vi "Setup UI temp.vi"(8 "error in (no error)":errorcluster, 10 "Set UI to input? (F)":bool, 11 "PC Reader.lvclass":refnum<class "PC Reader.lvclass">) -> (0 "error out":errorcluster, 3 "PC Reader out":refnum<class "PC Reader.lvclass">)   [LabVIEW 2009, in "PC Reader.lvclass"]
doc: "Setup UI (re)constructs an object -- populates its member data -- from a front panel the user can see. The VI should be as simple as possible so that a UI loop can poll it continuously for updates. \n\nThe VI is designed to be used as a subPanel within another VI. Wire true to \"Set UI to input\" only on the first call, just after inserting this VI into a subPanel, to populate its controls with the class's current values.\n\nSetup UI is distinct from the class constructor. Class constructors are not polymorphic, yet configure dialogs need to configure objects without knowing their type -- and polymorphism is the necessary solution. Thus, Setup UI is a polymorphic class constructor. This continously polled \"Setup UI\" concept is a kludge: a better idea would be an XControl, but those require a steeper learning curve."
uses:
  PC Reader.lvclass
  PC Reader.lvclass/PC Reader.ctl
panel:
  in  "template: Ch A sweep":bool
  in  "template: Ch A/B split":bool
  in  "template: continuous scan":bool
  in  "Gate B Ref":enum16{"t=0", "t=T/4", "t=T/2", "t=3T/4"}(ring)
  in  "Gate A Ref":enum16{"t=0", "t=T/4", "t=T/2", "t=3T/4"}(ring)
  out "Gate B Delay Actual":dbl[unit]
  out "Gate A Delay Actual":dbl[unit]
  in  "start vs mid. of gate":bool caption="Delays measured to"
  in  "Gate B %":dbl
  in  "Gate A %":dbl
  in  "time vs percent":bool caption="Width in"
  out "Gate B Mode":enum16{"CW", "Fixed", "Scan"}(ring)
  out "Gate A Mode":enum16{"CW", "Fixed", "Scan"}(ring)
  in  "Gate B Width":dbl[unit]
  in  "Gate B Delay":dbl[unit]
  in  "Gate A Delay":dbl[unit]
  in  "Gate A Width":dbl[unit]
  in  "Ext. Trigger?":bool
  in  "Ext. Trig. Freq.":dbl[unit]
  in  "Count Time":dbl[unit] format="%#_4g"
  in  "Send first pt to PC":bool
  in  "indAw?":bool
  in  "indAd?":bool
  in  "indBw?":bool
  in  "indBd?":bool
  # "Photon Counter Setup"
  # "Track ind.var.?\n(assumes in ns)"
  # "(PEM = 42.0762 kHz)"
  # "(If tracking, these times represent \nthe values for the first pt.)"
  # "PURE VIRTUAL\nMETHOD CALLED!"
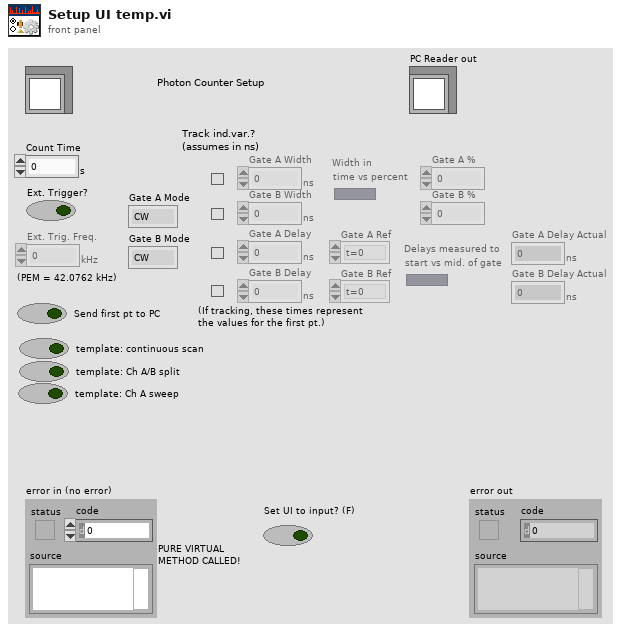
[diagram p1: front panel]
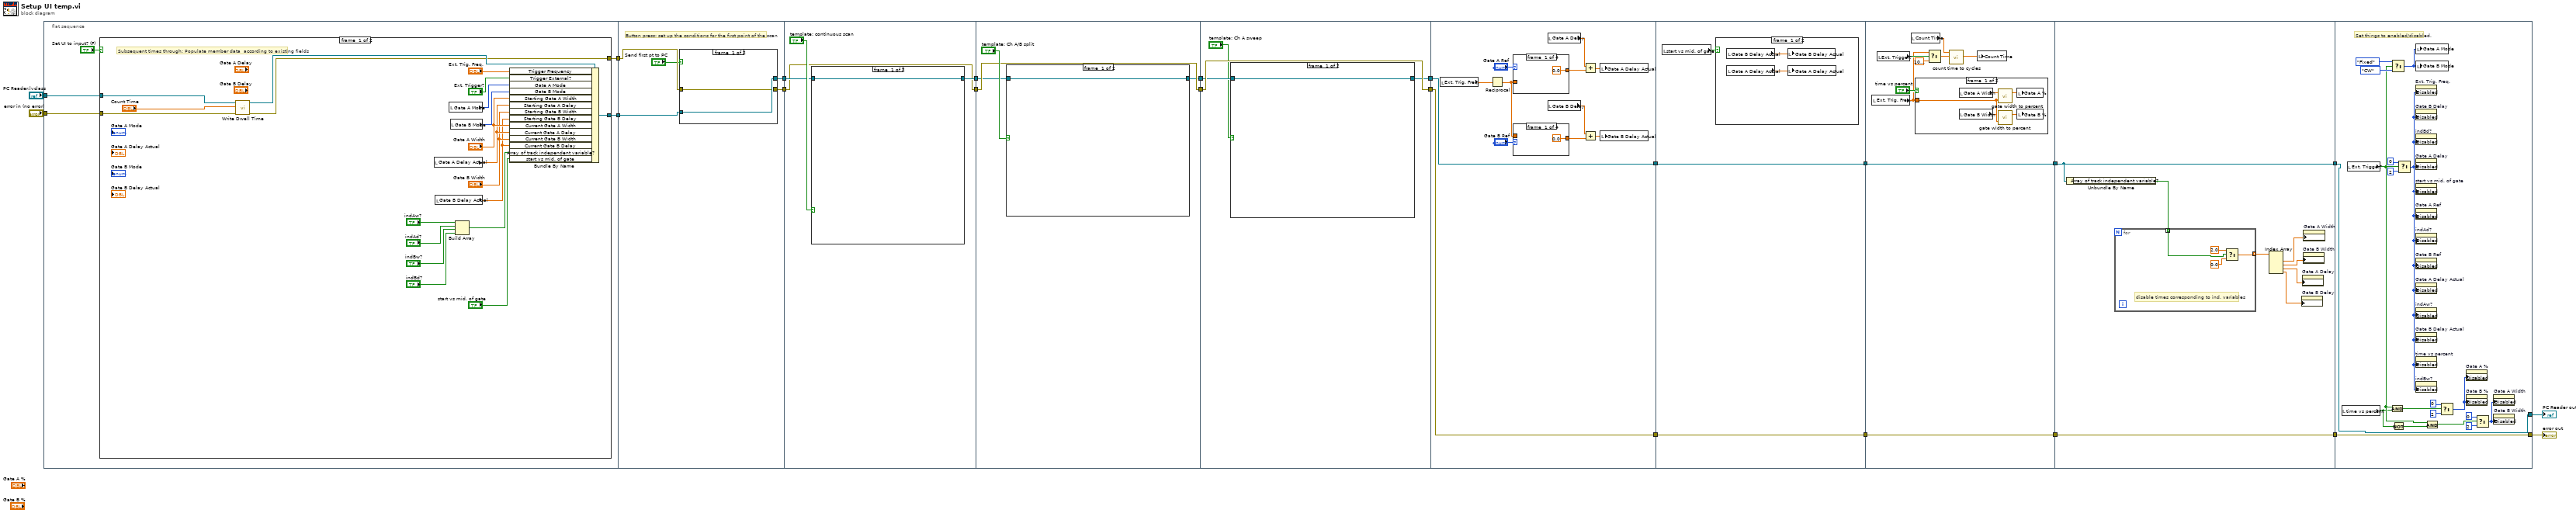
[diagram p0: block diagram]
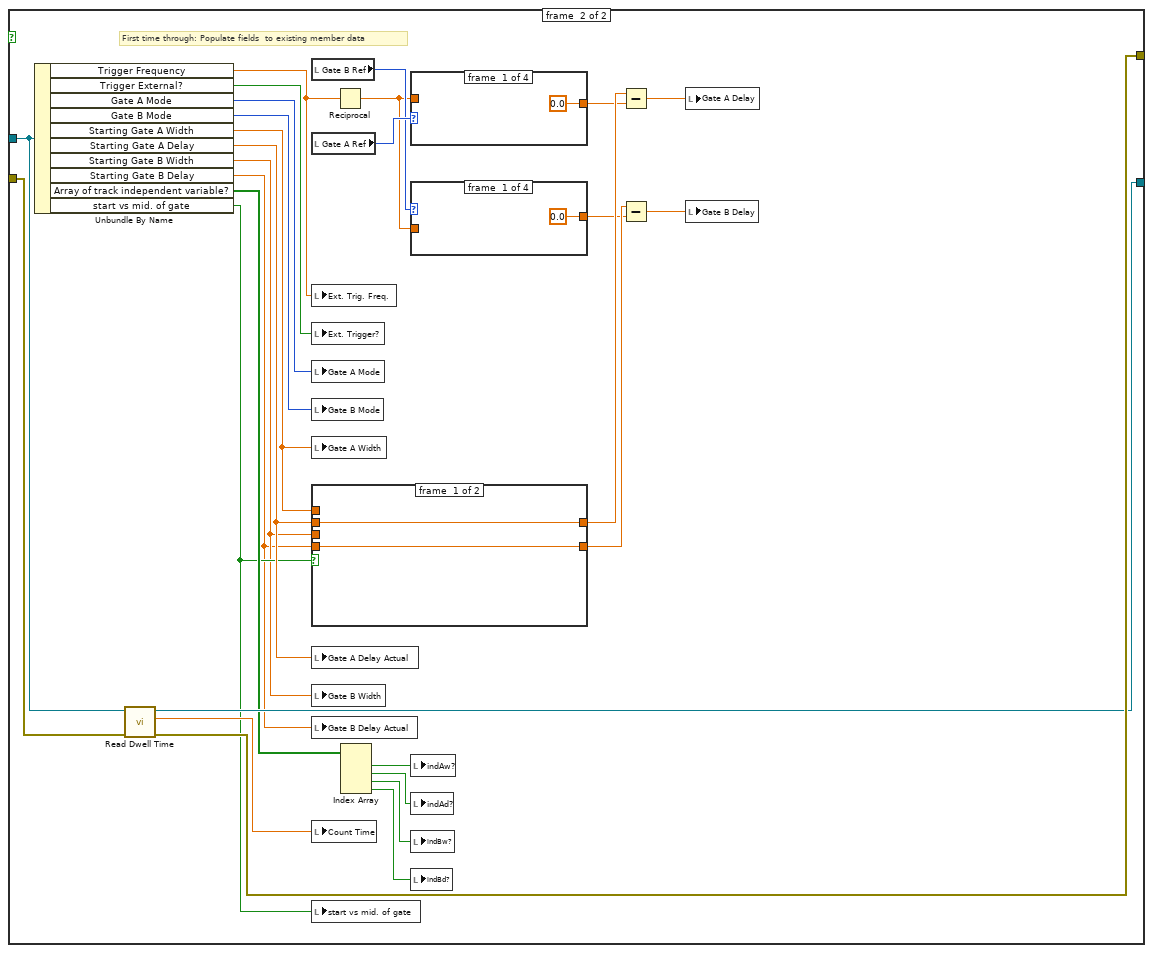
[diagram p2: hidden frame]
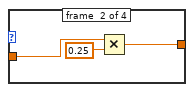
[diagram p3: hidden frame]
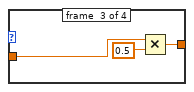
[diagram p4: hidden frame]
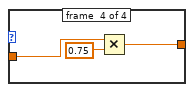
[diagram p5: hidden frame]
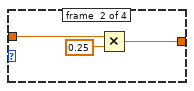
[diagram p6: hidden frame]
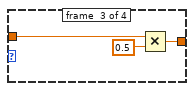
[diagram p7: hidden frame]
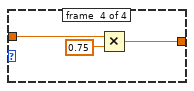
[diagram p8: hidden frame]
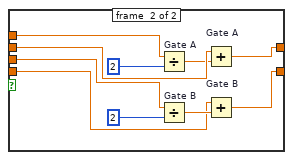
[diagram p9: hidden frame]
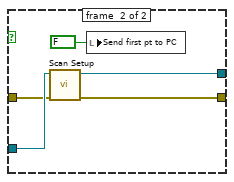
[diagram p10: hidden frame]
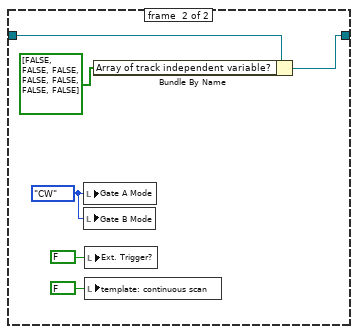
[diagram p11: hidden frame]
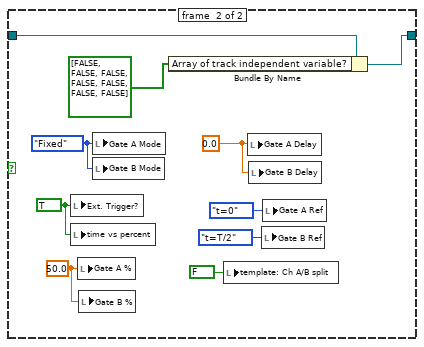
[diagram p12: hidden frame]
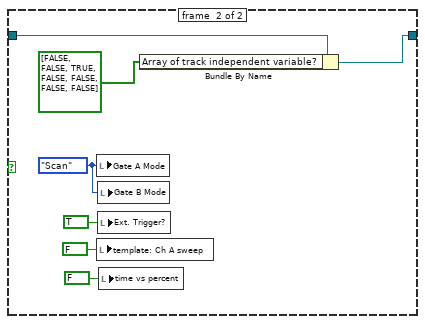
[diagram p13: hidden frame]
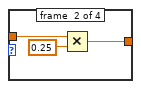
[diagram p14: hidden frame]
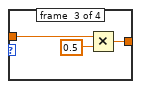
[diagram p15: hidden frame]
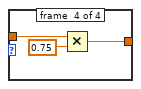
[diagram p16: hidden frame]
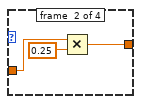
[diagram p17: hidden frame]
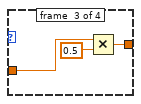
[diagram p18: hidden frame]
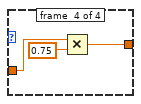
[diagram p19: hidden frame]
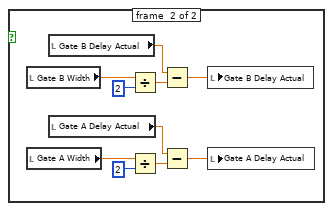
[diagram p20: hidden frame]
diagram:
  n1 = flat-sequence {
    tunnel: "error in (no error)" -> [w24]
    tunnel: [w27] -> w16
    tunnel: [w23] -> w15
    tunnel: "PC Reader.lvclass" -> [w25]
    tunnel: w16 -> [w112]
    tunnel: w15 -> [w111]
    tunnel: [w110] -> w14
    tunnel: [w108] -> w13
    tunnel: w14 -> [w120]
    tunnel: w13 -> [w122]
    tunnel: [w121] -> w12
    tunnel: [w120] -> w11
    tunnel: w12 -> [w132]
    tunnel: [w131] -> w10
    tunnel: w11 -> [w133]
    tunnel: [w133] -> w8
    tunnel: w10 -> [w148]
    tunnel: [w147] -> w9
    tunnel: w8 -> [w149]
    tunnel: [w149] -> w7
    tunnel: [w169] -> w19
    tunnel: [w168] -> w18
    tunnel: w9 -> [w168]
    tunnel: w7 -> [w169]
    tunnel: w19 -> [w192]
    tunnel: [w192] -> w21
    tunnel: w18 -> [w191]
    tunnel: [w191] -> w20
    tunnel: w21 -> [w213]
    tunnel: [w213] -> w6
    tunnel: w20 -> [w212]
    tunnel: [w212] -> w4
    tunnel: w6 -> [w231]
    tunnel: [w231] -> w5
    tunnel: w4 -> [w225]
    tunnel: [w225] -> w3
    tunnel: w5 -> [w237]
    tunnel: w3 -> [w236]
    tunnel: [w237] -> w2
    tunnel: [w236] -> w1
    frame #0 {
      n2 = case shown="True" "Set UI to input? (F)" {
        tunnel: [w39 w66] -> w27
        tunnel: w25 -> [w40 w67]
        tunnel: [w36 w68] -> w23
        tunnel: w24 -> [w35 w69]
        frame #0 {
          # "Subsequent times through: Populate member data  according to existing fields"
          n3 = call-dynamic "Write Dwell Time.vi"("error in (no error)"=w35, "Dwell Time"="Count Time", "Reader.lvclass in"=w40) -> ("error out"=w36:errorcluster, "Reader.lvclass out"=w38:refnum<class "PC Reader.lvclass">)  [unwired: 7 out]
          n4 = local read "Gate A Delay Actual"() -> (w32:dbl[unit])
          n5 = local read "Gate B Delay Actual"() -> (w30:dbl[unit])
          n6 = local read "Gate A Mode"() -> (w41:enum16{"CW", "Fixed", "Scan"})
          n7 = local read "Gate B Mode"() -> (w34:enum16{"CW", "Fixed", "Scan"})
          n8 = Build Array("indAw?", "indAd?", "indBw?", "indBd?") -> (w29:bool[])
          n9 = Bundle By Name(cluster=w38, "Trigger Frequency"="Ext. Trig. Freq.", "Trigger External?"="Ext. Trigger?", "Gate A Mode"=w41, "Gate B Mode"=w34, "Starting Gate A Width"="Gate A Width", "Starting Gate A Delay"=w32, "Starting Gate B Width"="Gate B Width", "Starting Gate B Delay"=w30, "Current Gate A Width"="Gate A Width", "Current Gate A Delay"=w32, "Current Gate B Width"="Gate B Width", "Current Gate B Delay"=w30, "Array of track independent variable?"=w29, "start vs mid. of gate"="start vs mid. of gate") -> (w39:refnum<class "PC Reader.lvclass">)
        }
        frame #1 {
          # "First time through: Populate fields  to existing member data"
          n10 = Unbundle By Name(w67) -> ("Trigger Frequency"=w62:dbl[unit], "Trigger External?"=w71:bool, "Gate A Mode"=w70:u16, "Gate B Mode"=w56:u16, "Starting Gate A Width"=w54:dbl[unit], "Starting Gate A Delay"=w55:dbl[unit], "Starting Gate B Width"=w51:dbl[unit], "Starting Gate B Delay"=w50:dbl[unit], "Array of track independent variable?"=w53:bool[], "start vs mid. of gate"=w52:bool)
          n11 = call-dynamic "Read Dwell Time.vi"("error in (no error)"=w69, "Reader.lvclass in"=w67) -> ("error out"=w68:errorcluster, "Dwell Time"=w65:dbl[unit], "Reader.lvclass out"=w66:refnum<class "PC Reader.lvclass">)  [unwired: 7 out]
          n12 = local read "Gate B Ref"() -> (w63:enum16{"t=0", "t=T/4", "t=T/2", "t=3T/4"})
          n13 = local read "Gate A Ref"() -> (w64:enum16{"t=0", "t=T/4", "t=T/2", "t=3T/4"})
          n14 = local write "Ext. Trig. Freq."(w62) -> ()
          n15 = local write "Ext. Trigger?"(w71) -> ()
          n16 = local write "Gate A Mode"(w70) -> ()
          n17 = local write "Gate B Mode"(w56) -> ()
          n18 = local write "Gate A Width"(w54) -> ()
          n19 = case shown="False" w52 {
            tunnel: [w97 w101] -> w60
            tunnel: w55 -> [w97 w105]
            tunnel: [w96 w100] -> w57
            tunnel: w54 -> [_ w102]
            tunnel: w51 -> [_ w99]
            tunnel: w50 -> [w96 w98]
            frame #0 {
            }
            frame #1 {
              n20 = Divide "Gate A"(x=w102, y=2) -> (x/y=w104:dbl[unit])
              n21 = Divide "Gate B"(x=w99, y=2) -> (x/y=w103:dbl[unit])
              n22 = Add "Gate A"(x=w105, y=w104) -> (x+y=w101:dbl[unit])
              n23 = Add "Gate B"(x=w98, y=w103) -> (x+y=w100:dbl[unit])
            }
          }
          n24 = local write "Gate A Delay Actual"(w55) -> ()
          n25 = local write "Gate B Width"(w51) -> ()
          n26 = local write "Gate B Delay Actual"(w50) -> ()
          n27 = local write "Count Time"(w65) -> ()
          n28 = local write "start vs mid. of gate"(w52) -> ()
          n29 = Reciprocal(x=w62) -> (1/x=w61:dbl[unit])
          n30 = Index Array(array=w53) -> (element #1=w72:bool, element #2=w73:bool, element #3=w74:bool, element #4=w75:bool)  [unwired: 4 in]
          n31 = case shown="\"t=T/4\"" w64 {
            tunnel: [dbl[unit] 0.0 ("x/y") w87 w90 w93] -> w59
            tunnel: w61 -> [_ w88 w91 w94]
            frame #0 {
            }
            frame #1 {
              n32 = Multiply(x=w88, y=0.25) -> (x*y=w87:dbl[unit])
            }
            frame #2 {
              n33 = Multiply(x=w91, y=0.5) -> (x*y=w90:dbl[unit])
            }
            frame #3 {
              n34 = Multiply(x=w94, y=0.75) -> (x*y=w93:dbl[unit])
            }
          }
          n35 = case shown="\"t=3T/4\"" w63 {
            tunnel: [dbl[unit] 0.0 ("x/y") w77 w80 w83] -> w48
            tunnel: w61 -> [_ w78 w81 w84]
            frame #0 {
            }
            frame #1 {
              n36 = Multiply(x=w78, y=0.25) -> (x*y=w77:dbl[unit])
            }
            frame #2 {
              n37 = Multiply(x=w81, y=0.5) -> (x*y=w80:dbl[unit])
            }
            frame #3 {
              n38 = Multiply(x=w84, y=0.75) -> (x*y=w83:dbl[unit])
            }
          }
          n39 = local write "indAw?"(w72) -> ()
          n40 = local write "indAd?"(w73) -> ()
          n41 = local write "indBw?"(w74) -> ()
          n42 = local write "indBd?"(w75) -> ()
          n43 = Subtract(x=w60, y=w59) -> (x-y=w58:dbl[unit])
          n44 = Subtract(x=w57, y=w48) -> (x-y=w49:dbl[unit])
          n45 = local write "Gate A Delay"(w58) -> ()
          n46 = local write "Gate B Delay"(w49) -> ()
        }
      }
    }
    frame #1 {
      # "Button press: set up the conditions for the first point of the scan"
      n47 = case shown="True" "Send first pt to PC" {
        tunnel: [w114 w115] -> w108
        tunnel: [w113 w116] -> w110
        tunnel: w112 -> [w114 w118]
        tunnel: w111 -> [w113 w117]
        frame #0 {
        }
        frame #1 {
          n48 = call-dynamic "Scan Setup.vi"("error in (no error)"=w117, "PC Reader in"=w118) -> ("error out"=w116:errorcluster, "PC Reader out"=w115:refnum<class "PC Reader.lvclass">)  [unwired: 8 out]
          n49 = local write "Send first pt to PC"(FALSE ("Send conds for first point to PG")) -> ()
        }
      }
    }
    frame #2 {
      n50 = case shown="True" "template: continuous scan" {
        tunnel: w122 -> [w124 w129]
        tunnel: [w124 w127] -> w121
        frame #0 {
        }
        frame #1 {
          w130 = enum16{"CW", "Fixed", "Scan"}."CW" ("Gate A Mode")
          n51 = local write "Gate A Mode"(w130) -> ()
          n52 = local write "Gate B Mode"(w130) -> ()
          n53 = local write "Ext. Trigger?"(FALSE ("Ext. Trigger?")) -> ()
          n54 = local write "template: continuous scan"(FALSE ("template: continuous scan")) -> ()
          n55 = Bundle By Name(cluster=w129, "Array of track independent variable?"=bool[] [FALSE, FALSE, FALSE, FALSE, FALSE, FALSE, FALSE]) -> (w127:refnum<class "PC Reader.lvclass">)
        }
      }
    }
    frame #3 {
      n56 = case shown="True" "template: Ch A/B split" {
        tunnel: w132 -> [w135 w145]
        tunnel: [w135 w144] -> w131
        frame #0 {
        }
        frame #1 {
          w139 = dbl[unit] 0.0 ("Gate A Delay")
          w140 = 50.0 ("Gate A %")
          w141 = TRUE ("Ext. Trigger?")
          w142 = enum16{"CW", "Fixed", "Scan"}."Fixed" ("Gate A Mode")
          n57 = local write "Ext. Trigger?"(w141) -> ()
          n58 = local write "time vs percent"(w141) -> ()
          n59 = local write "Gate A %"(w140) -> ()
          n60 = local write "Gate B %"(w140) -> ()
          n61 = local write "Gate A Mode"(w142) -> ()
          n62 = local write "Gate B Mode"(w142) -> ()
          n63 = Bundle By Name(cluster=w145, "Array of track independent variable?"=bool[] [FALSE, FALSE, FALSE, FALSE, FALSE, FALSE, FALSE]) -> (w144:refnum<class "PC Reader.lvclass">)
          n64 = local write "template: Ch A/B split"(FALSE ("template: Ch A/B split")) -> ()
          n65 = local write "Gate A Delay"(w139) -> ()
          n66 = local write "Gate B Delay"(w139) -> ()
          n67 = local write "Gate B Ref"(enum16{"t=0", "t=T/4", "t=T/2", "t=3T/4"}."t=T/2" ("Gate B Ref")) -> ()
          n68 = local write "Gate A Ref"(enum16{"t=0", "t=T/4", "t=T/2", "t=3T/4"}."t=0" ("Gate A Ref")) -> ()
        }
      }
    }
    frame #4 {
      n69 = case shown="True" "template: Ch A sweep" {
        tunnel: w148 -> [w150 w157]
        tunnel: [w150 w156] -> w147
        frame #0 {
        }
        frame #1 {
          w154 = enum16{"CW", "Fixed", "Scan"}."Scan" ("Gate A Mode")
          n70 = local write "Gate A Mode"(w154) -> ()
          n71 = local write "template: Ch A sweep"(FALSE ("template: Ch A sweep")) -> ()
          n72 = local write "Gate B Mode"(w154) -> ()
          n73 = local write "Ext. Trigger?"(TRUE ("Ext. Trigger?")) -> ()
          n74 = local write "time vs percent"(FALSE ("time vs percent")) -> ()
          n75 = Bundle By Name(cluster=w157, "Array of track independent variable?"=bool[] [FALSE, FALSE, TRUE, FALSE, FALSE, FALSE, FALSE]) -> (w156:refnum<class "PC Reader.lvclass">)
        }
      }
    }
    frame #5 {
      n76 = local read "Ext. Trig. Freq."() -> (w165:dbl[unit])
      n77 = Reciprocal(x=w165) -> (1/x=w164:dbl[unit])
      n78 = case shown="\"t=0\", Default" "Gate A Ref" {
        tunnel: w164 -> [_ w182 w185 w188]
        tunnel: [dbl[unit] 0.0 ("x/y") w181 w184 w187] -> w162
        frame #0 {
        }
        frame #1 {
          n79 = Multiply(x=w182, y=0.25) -> (x*y=w181:dbl[unit])
        }
        frame #2 {
          n80 = Multiply(x=w185, y=0.5) -> (x*y=w184:dbl[unit])
        }
        frame #3 {
          n81 = Multiply(x=w188, y=0.75) -> (x*y=w187:dbl[unit])
        }
      }
      n82 = case shown="\"t=T/4\"" "Gate B Ref" {
        tunnel: w164 -> [_ w172 w175 w178]
        tunnel: [dbl[unit] 0.0 ("x/y") w171 w174 w177] -> w159
        frame #0 {
        }
        frame #1 {
          n83 = Multiply(x=w172, y=0.25) -> (x*y=w171:dbl[unit])
        }
        frame #2 {
          n84 = Multiply(x=w175, y=0.5) -> (x*y=w174:dbl[unit])
        }
        frame #3 {
          n85 = Multiply(x=w178, y=0.75) -> (x*y=w177:dbl[unit])
        }
      }
      n86 = local read "Gate A Delay"() -> (w163:dbl[unit])
      n87 = local read "Gate B Delay"() -> (w160:dbl[unit])
      n88 = Add(x=w163, y=w162) -> (x+y=w161:dbl[unit])
      n89 = Add(x=w160, y=w159) -> (x+y=w158:dbl[unit])
      n90 = local write "Gate A Delay Actual"(w161) -> ()
      n91 = local write "Gate B Delay Actual"(w158) -> ()
    }
    frame #6 {
      n92 = local read "start vs mid. of gate"() -> (w190:bool)
      n93 = case shown="True" w190 {
        frame #0 {
          n94 = local read "Gate B Delay Actual"() -> (w193:dbl[unit])
          n95 = local read "Gate A Delay Actual"() -> (w194:dbl[unit])
          n96 = local write "Gate B Delay Actual"(w193) -> ()
          n97 = local write "Gate A Delay Actual"(w194) -> ()
        }
        frame #1 {
          n98 = local read "Gate B Width"() -> (w197:dbl[unit])
          n99 = local read "Gate A Width"() -> (w201:dbl[unit])
          n100 = local read "Gate B Delay Actual"() -> (w198:dbl[unit])
          n101 = local read "Gate A Delay Actual"() -> (w202:dbl[unit])
          n102 = Divide(x=w197, y=2) -> (x/y=w199:dbl[unit])
          n103 = Divide(x=w201, y=2) -> (x/y=w200:dbl[unit])
          n104 = Subtract(x=w198, y=w199) -> (x-y=w195:dbl[unit])
          n105 = Subtract(x=w202, y=w200) -> (x-y=w196:dbl[unit])
          n106 = local write "Gate B Delay Actual"(w195) -> ()
          n107 = local write "Gate A Delay Actual"(w196) -> ()
        }
      }
    }
    frame #7 {
      n108 = local read "Ext. Trig. Freq."() -> (w208:dbl[unit])
      n109 = local read "Ext. Trigger?"() -> (w209:bool)
      n110 = local read "Count Time"() -> (w210:dbl[unit])
      n111 = case shown="True" "time vs percent" {
        tunnel: w208 -> [w218 w221]
        frame #0 {
          n112 = local read "Gate A Width"() -> (w217:dbl[unit])
          n113 = local read "Gate B Width"() -> (w216:dbl[unit])
          n114 = call "gate width to percent.vi"("Trigger Freq"=w218, "Gate width"=w217) -> ("Gate %"=w215:dbl)  [unwired: 1 out]
          n115 = call "gate width to percent.vi"("Trigger Freq"=w218, "Gate width"=w216) -> ("Gate %"=w214:dbl)  [unwired: 1 out]
          n116 = local write "Gate A %"(w215) -> ()
          n117 = local write "Gate B %"(w214) -> ()
        }
        frame #1 {
          n118 = local read "Gate B %"() -> (w219:dbl)
          n119 = local read "Gate A %"() -> (w220:dbl)
          n120 = call "gate percent to width.vi"("Trigger Freq"=w221, "Gate %"=w219) -> ("Gate width"=w223:dbl[unit])  [unwired: 1 out]
          n121 = call "gate percent to width.vi"("Trigger Freq"=w221, "Gate %"=w220) -> ("Gate width"=w222:dbl[unit])  [unwired: 1 out]
          n122 = local write "Gate B Width"(w223) -> ()
          n123 = local write "Gate A Width"(w222) -> ()
        }
      }
      n124 = Select(t=w208, s=w209, f=dbl[unit] 10000000.0 ("Trigger Freq")) -> (s? t:f=w206:dbl[unit])
      n125 = call "count time to cycles.vi"("Trigger Freq"=w206, "Count Time Set"=w210) -> ("Count Time Current"=w205:dbl[unit])  [unwired: 1 in, 4 out]
      n126 = local write "Count Time"(w205) -> ()
    }
    frame #8 {
      n127 = Unbundle By Name(w225) -> ("Array of track independent variable?"=w224:bool[])
      n128 = for {
        tunnel: [w233] -> w226 mode=indexing
        tunnel: w224 -> [w232] mode=indexing
        # "disable times corresponding to ind. variables"
        n129 = Select(t=2.0, s=w232, f=0.0) -> (s? t:f=w233:dbl)
      }
      n130 = Index Array(array=w226) -> (element #1=w227:dbl, element #2=w228:dbl, element #3=w229:dbl, element #4=w230:dbl)  [unwired: 4 in]
      n131 = property on="Gate B Delay" class="DigNum (strict)"("DisabledEnum"=w230) -> ()  [unwired: 2 in, 2 out]
      n132 = property on="Gate A Delay" class="DigNum (strict)"("DisabledEnum"=w229) -> ()  [unwired: 2 in, 2 out]
      n133 = property on="Gate B Width" class="DigNum (strict)"("DisabledEnum"=w228) -> ()  [unwired: 2 in, 2 out]
      n134 = property on="Gate A Width" class="DigNum (strict)"("DisabledEnum"=w227) -> ()  [unwired: 2 in, 2 out]
    }
    frame #9 {
      # "Set things to enabled/disabled."
      n135 = local read "time vs percent"() -> (w239:bool)
      n136 = local read "Ext. Trigger?"() -> (w240:bool)
      n137 = And(x=w240, y=w239) -> (x .and. y?=w247:bool)
      n138 = Select(t=enum16{"CW", "Fixed", "Scan"}."Fixed" ("Gate A Mode"), s=w240, f=enum16{"CW", "Fixed", "Scan"}."CW" ("Gate A Mode")) -> (s? t:f=w252:enum16{"CW", "Fixed", "Scan"})
      n139 = Not(x=w239) -> (.not. x?=w241:bool)
      n140 = Select(t=0, s=w240, f=2) -> (s? t:f=w238:i32)
      n141 = local write "Gate A Mode"(w252) -> ()
      n142 = local write "Gate B Mode"(w252) -> ()
      n143 = property on="Ext. Trig. Freq." class="DigNum (strict)"("Disabled"=w238) -> ()  [unwired: 2 in, 2 out]
      n144 = property on="Gate B Delay" class="DigNum (strict)"("Disabled"=w238) -> ()  [unwired: 2 in, 2 out]
      n145 = property on="indBd?" class="Bool (strict)"("Disabled"=w238) -> ()  [unwired: 2 in, 2 out]
      n146 = property on="Gate A Delay" class="DigNum (strict)"("Disabled"=w238) -> ()  [unwired: 2 in, 2 out]
      n147 = property on="start vs mid. of gate" class="Bool (strict)"("Disabled"=w238) -> ()  [unwired: 2 in, 2 out]
      n148 = property on="Gate A Ref" class="Enum (strict)"("Disabled"=w238) -> ()  [unwired: 2 in, 2 out]
      n149 = property on="indAd?" class="Bool (strict)"("Disabled"=w238) -> ()  [unwired: 2 in, 2 out]
      n150 = property on="Gate B Ref" class="Enum (strict)"("Disabled"=w238) -> ()  [unwired: 2 in, 2 out]
      n151 = property on="Gate A Delay Actual" class="DigNum (strict)"("Disabled"=w238) -> ()  [unwired: 2 in, 2 out]
      n152 = property on="indAw?" class="Bool (strict)"("Disabled"=w238) -> ()  [unwired: 2 in, 2 out]
      n153 = property on="Gate B Delay Actual" class="DigNum (strict)"("Disabled"=w238) -> ()  [unwired: 2 in, 2 out]
      n154 = property on="time vs percent" class="Bool (strict)"("Disabled"=w238) -> ()  [unwired: 2 in, 2 out]
      n155 = property on="indBw?" class="Bool (strict)"("Disabled"=w238) -> ()  [unwired: 2 in, 2 out]
      n156 = And(x=w240, y=w241) -> (x .and. y?=w243:bool)
      n157 = Select(t=0, s=w247, f=2) -> (s? t:f=w246:i32)
      n158 = property on="Gate A %" class="DigNum (strict)"("Disabled"=w246) -> ()  [unwired: 2 in, 2 out]
      n159 = property on="Gate B %" class="DigNum (strict)"("Disabled"=w246) -> ()  [unwired: 2 in, 2 out]
      n160 = Select(t=0, s=w243, f=2) -> (s? t:f=w242:i32)
      n161 = property on="Gate A Width" class="DigNum (strict)"("Disabled"=w242) -> ()  [unwired: 2 in, 2 out]
      n162 = property on="Gate B Width" class="DigNum (strict)"("Disabled"=w242) -> ()  [unwired: 2 in, 2 out]
    }
  }
  "error out" <- w2
  "PC Reader out" <- w1
